vi "Area Scoring.vi"(10 "Convex Hull Area":dbl, 11 "Area":dbl) -> (3 "Score":dbl)   [LabVIEW 2025]
doc: "Calculate a score based on area and convex hull area. Convex hull area fills holes and convex areas of the shape. It is equivalent to putting a rubber band around the shape and computing the area enclosed by the band."
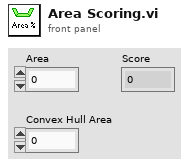
[diagram p1: front panel]
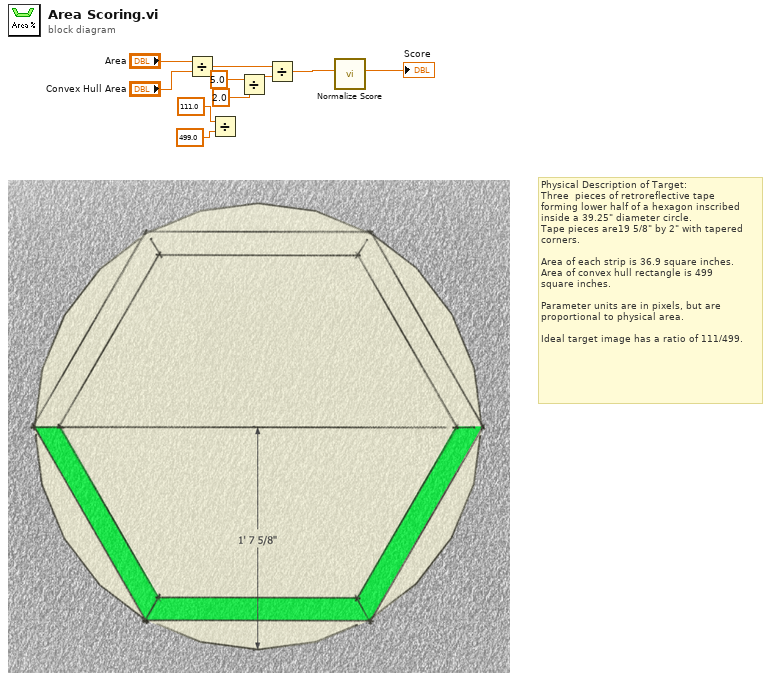
[diagram p0: block diagram]
diagram:
  # "Physical Description of Target:\nThree  pieces of retroreflective tape\nforming lower half of a hexagon inscribed\ninside a 39.25\" diameter circle.\nTape pieces are19 5/8\" by 2\" with tapered\ncorners.\n\nArea of each strip is 36.9 square inches.\nArea of convex hull rectangle is 499\nsquare inches.\n\nParameter units are in pixels, but are\nproportional to physical area.\n\nIdeal target image has a ratio of 111/499."
  n1 = Divide(x="Area", y="Convex Hull Area") -> (x/y=w9:dbl)
  n2 = Divide(x=111.0 ("length"), y=499.0 ("length")) -> ()  [unwired: 1 out]
  n3 = Divide(x=5.0, y=2.0) -> (x/y=w3:dbl)
  n4 = Divide(x=w9, y=w3) -> (x/y=w7:dbl)
  n5 = call "Normalize Score.vi"("Value"=w7) -> ("Score"=→"Score":dbl)  [unwired: 10 in]
